vi "LINX - PmodCMPS.vi"() -> ()   [LabVIEW 2019]
doc: "PmodCMPS\n\nThis example demonstrates how to read the angular velocity values from the CMPS.\n\nInstructions:\n1. Select the COM Port associated with the LINX device\n2. Select the I2C Channel that the Pmod is connected to.\n3. Click the Run Arrow."
uses:
  <vilib>/MakerHub/LINX/LMH-LINX.lvlib
  <vilib>/MakerHub/LINX/Public/Sensors/Pmods/CMPS/PmodCMPS.lvlib
panel:
  out "Waveform Chart":T1(graph)
  out "Gauss":cluster{"X":dbl, "Y":dbl, "Z":dbl}
  in  "Stop Button":bool
  in  "Serial Port":refnum<visa-resource-name>="N/A"
  in  "I2C Channel (0)":u8
  # "PmodCMPS\n\nThis example demonstrates how to read the angular velocity values from the CMPS.\n\nInstructions:\n1. Select the COM Port associated with the LINX device\n2. Select the I2C Channel that the Pmod is connected to.\n3. Click the Run Arrow."
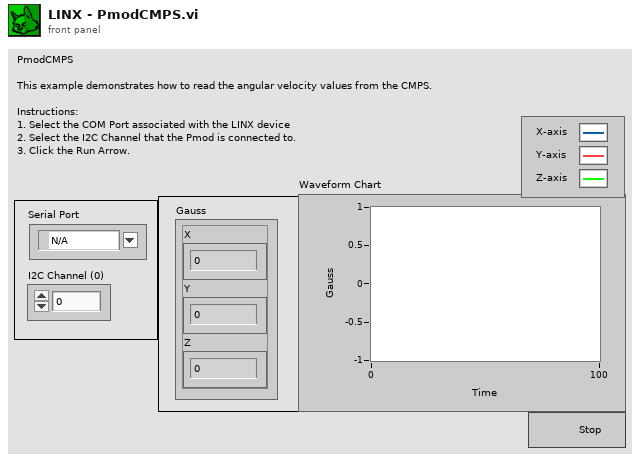
[diagram p1: front panel]
types:
  T1 = cluster{"Decimal I16":dbl, "Decimal I16":dbl, "Decimal I16":dbl}
  T2 = typedef "LMH-LINX.lvlib/LINX Ref.ctl" = cluster{"IO":T3, "Interface":T4, "LINX Device Config":T5}
  T3 = typedef "LMH-LINX.lvlib/Platform.ctl" = enum16{"Remote", "Local"}
  T4 = typedef "LMH-LINX.lvlib/Interface.ctl" = enum16{"Serial", "TCP"}
  T5 = typedef "LMH-LINX.lvlib/Device.lvlib/LINX Device Config.ctl" = cluster{"Interface":T4, "COM Port":refnum<visa-resource-name>, "TCP Configuration":T6, "Device Family":u8, "Device ID":u8, "Device Name":string, "TCP Ref":refnum<k5>, "Channels":T7}
  T6 = typedef "LMH-LINX.lvlib/Device.lvlib/TCP Config.ctl" = cluster{"IP Address":string, "Port":u16}
  T7 = typedef "LMH-LINX.lvlib/Channels.ctl" = cluster{"DI":u8[], "DO":u8[], "AI":u8[], "AO":u8[], "PWM":u8[], "QE":u8[], "UART":u8[], "I2C 2":u8[], "SPI":u8[], "CAN":u8[], "Servo":u8[], "AI Ref (V)":dbl, "AI Resolution (Bits)":u8, "AO Ref (V)":dbl, "AO Resolution (Bits)":u8}
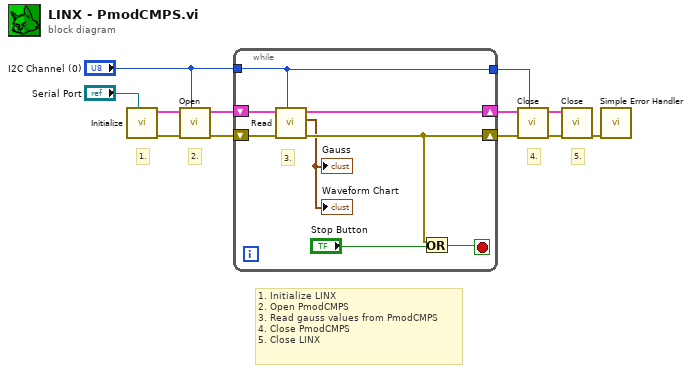
[diagram p0: block diagram]
diagram:
  # "1. Initialize LINX\n2. Open PmodCMPS\n3. Read gauss values from PmodCMPS\n4. Close PmodCMPS\n5. Close LINX"
  # "5."
  # "4."
  # "2."
  # "1."
  n1 = call <vilib>:"Initialize.vi"("Serial Port"="Serial Port") -> ("Error Out"=w10:errorcluster, "LINX Resource"=w11:T2)  [unwired: 8 in, 1 out]
  n2 = call <vilib>:"Open.vi"("I2C Channel (0)"="I2C Channel (0)", "Error In"=w10, "LINX Resource"=w11) -> ("Error Out"=w4:errorcluster, "LINX Resource"=w5:T2)  [unwired: 7 in]
  n3 = while {
    shift-right: [w17] -> w1
    shift-left: w5 -> [w14]
    shift-right: [w16] -> w8
    shift-left: w4 -> [w20]
    tunnel: "I2C Channel (0)" -> [w13]
    tunnel: [w13] -> w2
    stop <- w18 stop-if-true
    # "3."
    n4 = call <vilib>:"Read.vi"("I2C Channel (0)"=w13, "Error In"=w20, "LINX Resource"=w14) -> ("Error Out"=w16:errorcluster, "Compass (Gauss)"=→"Gauss" →"Waveform Chart":cluster{"X":dbl, "Y":dbl, "Z":dbl}, "LINX Resource"=w17:T2)  [unwired: 6 in]
    n5 = Or(x=w16, y="Stop Button") -> (x .or. y?=w18:bool)
  }
  n6 = call <vilib>:"Close.vi"("I2C Channel (0)"=w2, "Error In"=w8, "LINX Resource"=w1) -> ("Error Out"=w6:errorcluster, "LINX Resource"=w7:T2)  [unwired: 7 in]
  n7 = call <vilib>:"Close.vi"("Error In"=w6, "LINX Resource"=w7) -> ("Error Out"=w9:errorcluster)  [unwired: 9 in]
  n8 = call <vilib>:"Simple Error Handler.vi"("error in (no error)"=w9) -> ()  [unwired: 4 in, 5 out]
